vi "FIFOBuffer.vi"(1 "Set/Get":bool, 2 "FIFOBuffer (input)":u32[](array[numeric])) -> (0 "FIFOBuffer (output)":u32[](array[numeric]))   [LabVIEW 2009]
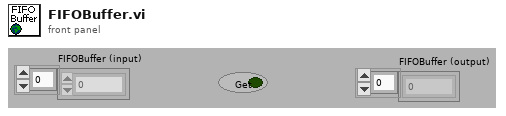
[diagram p1: front panel]
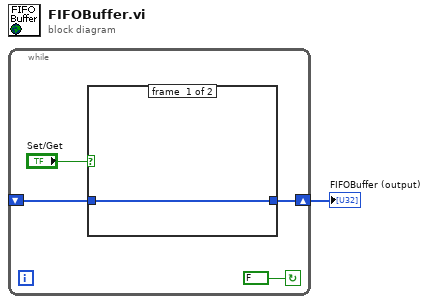
[diagram p0: block diagram]
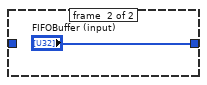
[diagram p2: hidden frame]
diagram:
  n1 = while {
    shift-right: [w4] -> w1
    shift-left: _ -> [w3]
    stop <- FALSE continue-if-true
    n2 = case shown="True" "Set/Get" {
      tunnel: [w6 "FIFOBuffer (input)"] -> w4
      tunnel: w3 -> [w6 _]
      frame #0 {
      }
      frame #1 {
      }
    }
  }
  "FIFOBuffer (output)" <- w1
